vi "choosePath.vi"(8 "error in (no error)":errorcluster, 11 "PixelflySettings in":refnum<class "PixelflySettings.lvclass">) -> (0 "error out":errorcluster, 1 "cancelled?":bool, 2 "Path":path, 3 "PixelflySettings out":refnum<class "PixelflySettings.lvclass">)   [LabVIEW 2011, in "Tools.lvlib" / "Settings.lvlib" / "PixelflySettings.lvclass"]
uses:
  PixelflySettings.lvclass
  Filing/FileSystem/FileSystem.lvclass
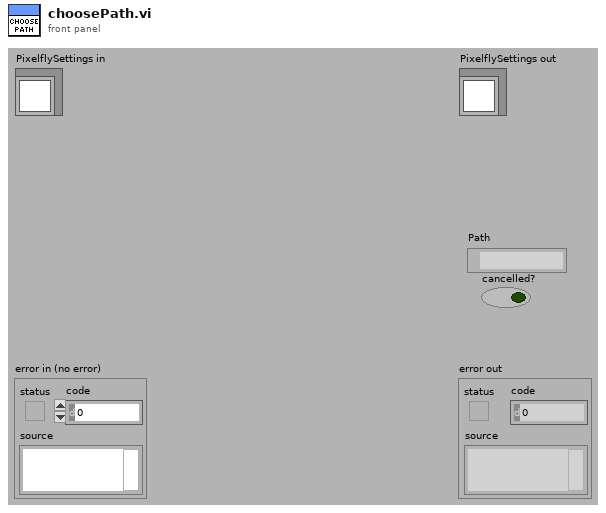
[diagram p1: front panel]
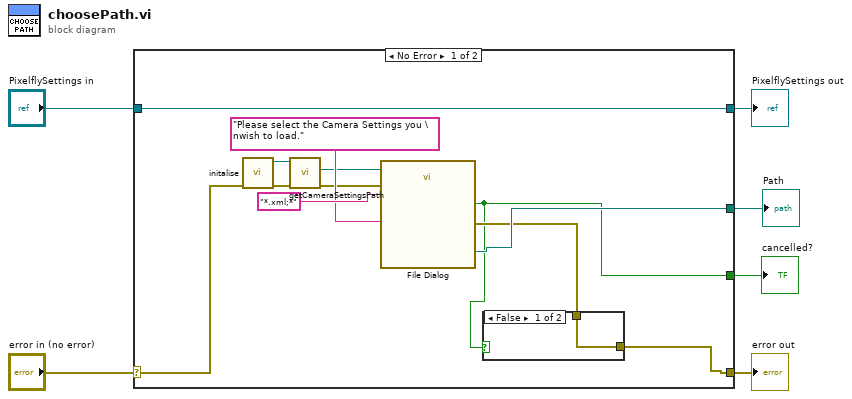
[diagram p0: block diagram]
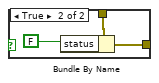
[diagram p2: hidden frame]
diagram:
  n1 = case shown="No Error" "error in (no error)" {
    selector: "error in (no error)" -> [w11 w24]
    tunnel: [w8 w24] -> w5
    tunnel: [w18 w23] -> w3
    tunnel: "PixelflySettings in" -> [w18 w23]
    tunnel: [w10 _] -> w2
    tunnel: [w7 _] -> w1
    frame No Error {
      n2 = call "initalise.vi"("error in (no error)"=w11) -> ("error out"=w14:errorcluster, "FileSystem out"=w15:refnum<class "FileSystem.lvclass">)  [unwired: 9 in]
      n3 = call-dynamic "getCameraSettingsPath.vi"("error in (no error)"=w14, "FileSystem.lvclass in"=w15) -> ("error out"=w12:errorcluster, "CameraSettingsPath"=w13:path)  [unwired: 7 in, 1 out]
      n4 = call "File Dialog"("start path"=w13, "prompt"="Please select the Camera Settings you \nwish to load.", "error in"=w12, "pattern (all files)"="*.xml;*") -> ("selected path"=w10:path, "cancelled"=w7:bool, "error out"=w9:errorcluster)  [unwired: 8 in, 1 out]
      n5 = case shown="False" w7 {
        tunnel: w9 -> [w19 w22]
        tunnel: [w19 w20] -> w8
        frame False {
        }
        frame True {
          n6 = Bundle By Name(cluster=w22, "status"=FALSE) -> (w20:errorcluster)
        }
      }
    }
    frame Error {
    }
  }
  "error out" <- w5
  "PixelflySettings out" <- w3
  "Path" <- w2
  "cancelled?" <- w1
